vi "RelinkFixToSerialNumber.vi"(0 "class data in":refnum<class "CMESAPI.lvclass">, 5 "serialNumber":string, 7 "equipment":string, 9 "WorkorderNumber":string, 11 "error in (no error)":errorcluster) -> (4 "class data out":refnum<class "CMESAPI.lvclass">, 15 "error out":errorcluster)   [LabVIEW 2020, in "CMESAPI.lvlib" / "CMESAPI.lvclass"]
uses:
  CMESAPI.lvclass
  <vilib>/gpm_packages/@cs/event-logger/Source/Composed Log/Types/Log Level.ctl
  CMESAPI.lvclass/CMESAPI.ctl
  C:/Users/Fred Guo/Desktop/API_Salcomp_CMES/Libraries/CMESAPI/CMESAPI_Fw4.0_1.9.2/CMESAPI.dll
  CMESAPI_Fw4.0_1.9.2/CMESAPI.dll
  <vilib>/gpm_packages/@cs/event-logger/Source/Composed Log/LoggerReference/LoggerReference.lvclass/LoggerReference.ctl
  <vilib>/gpm_packages/@cs/event-logger/Source/Composed Log/LoggerReference/Log.vi
  <vilib>/gpm_packages/@cs/event-logger/Source/Composed Log/LoggerReference/Get Valid Event Time.vi
  <vilib>/gpm_packages/@cs/event-logger/Source/Composed Log/LoggerReference/Remove Stale Logs.vi
  <vilib>/gpm_packages/@cs/event-logger/Source/Composed Log/LoggerReference/LoggerReference.lvclass
  <vilib>/gpm_packages/@cs/event-logger/Source/Composed Log/Composed Log.lvlib
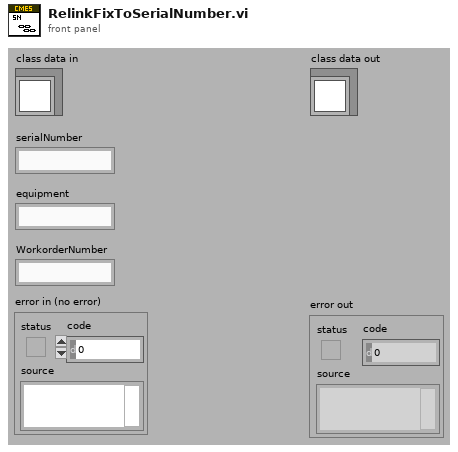
[diagram p1: front panel]
types:
  T1 = typedef "Composed Log.lvlib/Log Level.ctl" = enum16{"Debug", "Info", "Warning", "Error", "Critical"}
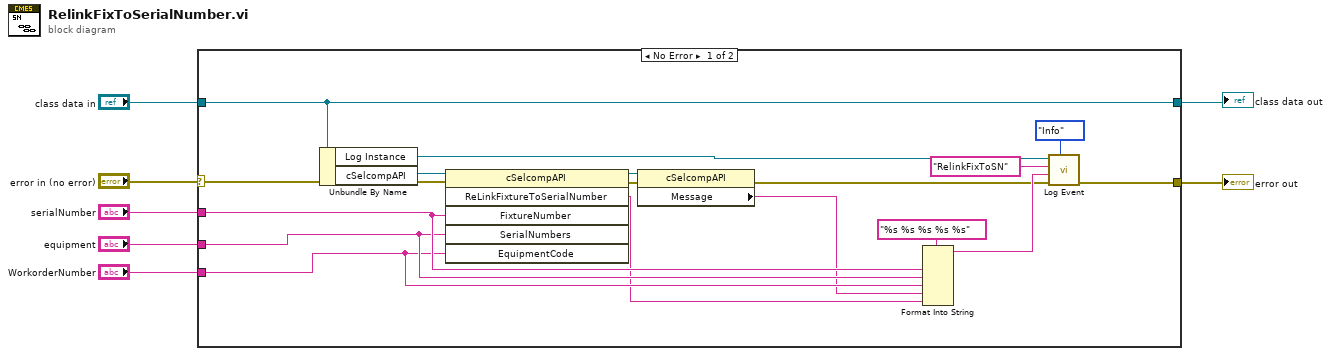
[diagram p0: block diagram]
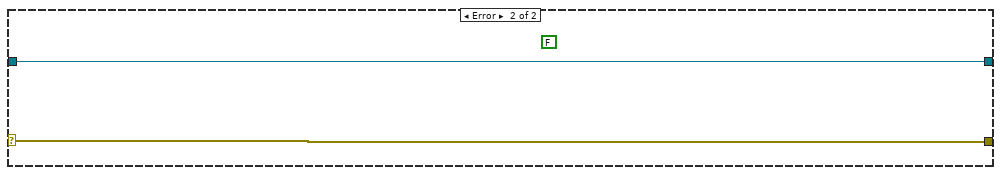
[diagram p2: hidden frame]
diagram:
  n1 = case shown="No Error" "error in (no error)" {
    selector: "error in (no error)" -> [w22 w26]
    tunnel: [w14 w26] -> w6
    tunnel: "class data in" -> [w24 w25]
    tunnel: [w24 w25] -> w4
    tunnel: "WorkorderNumber" -> [w11 _]
    tunnel: "equipment" -> [w12 _]
    tunnel: "serialNumber" -> [w13 _]
    frame No Error {
      n2 = Unbundle By Name(w24) -> ("Log Instance"=w9:refnum<class "LoggerReference.lvclass">, "cSelcompAPI"=w23:refnum<k24>)
      n3 = invoke on="Invoke Node" class="cSelcompAPI" method="ReLinkFixtureToSerialNumber"(reference=w23, error in=w22, "FixtureNumber"=w13, "SerialNumbers"=w12, "EquipmentCode"=w11) -> (reference out=w21:refnum<k24>, error out=w20:errorcluster, "ReLinkFixtureToSerialNumber"=w8:string)  [unwired: 1 in, 3 out]
      n4 = property class="cSelcompAPI"(reference=w21, error in=w20) -> (error out=w15:errorcluster, "Message"=w10:string)  [unwired: 1 out]
      n5 = Format Into String(format string="%s %s %s %s %s", w13, w12, w11, w10, w8) -> (resulting string=w17:string)  [unwired: 2 in, 1 out]
      n6 = call <vilib>:"Log Event.vi"("Event Level"=Log_Level."Info", "error in (no error)"=w15, "Data To Log"=w17, "SourceID"="RelinkFixToSN", "Log Instance"=w9) -> ("error out"=w14:errorcluster)  [unwired: 5 in, 1 out]
    }
    frame Error {
      (unwired) FALSE ("CheckRouteForSerialNumber")
    }
  }
  "error out" <- w6
  "class data out" <- w4
